vi "Convert To Palette Data.vi"(8 "error in (no error)":errorcluster, 11 "Predicted Data[]":string[](array[string])) -> (0 "error out":errorcluster, 3 "Array":T1[](array[typedef]))   [LabVIEW 2014, in "SmartPalette.lvlib"]
uses:
  SmartPalette.lvlib
  Controls/Palette Data.ctl
  <vilib>/picture/picture.llb/imagedata.ctl
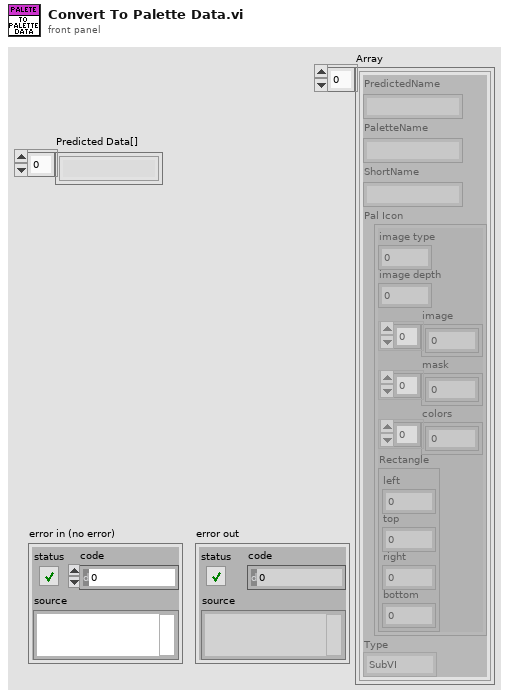
[diagram p1: front panel]
types:
  T1 = typedef "SmartPalette.lvlib/Palette Data.ctl" = cluster{"PredictedName":string, "PaletteName":string, "ShortName":string, "Pal Icon":T2, "Type":enum16{"SubVI", "Function"}}
  T2 = typedef "imagedata.ctl" = cluster{"image type":i32, "image depth":i32, "image":u8[], "mask":u8[], "colors":u32[], "Rectangle":cluster{"left":i16, "top":i16, "right":i16, "bottom":i16}}
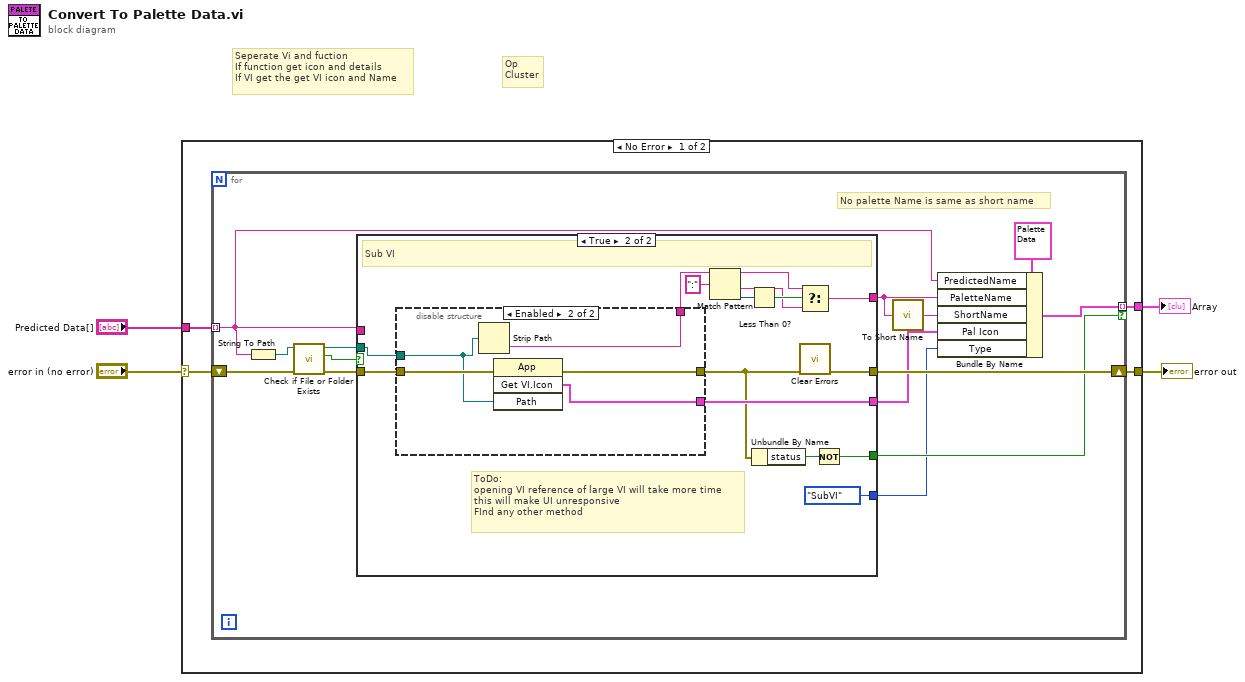
[diagram p0: block diagram]
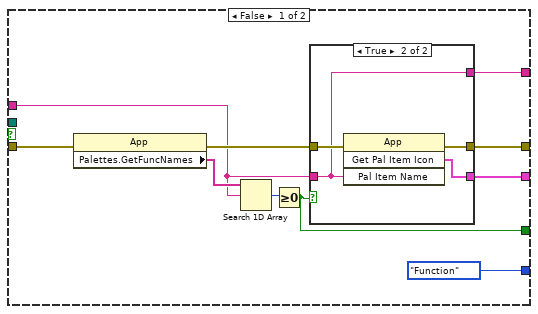
[diagram p2: hidden frame]
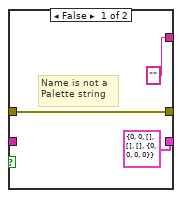
[diagram p3: hidden frame]
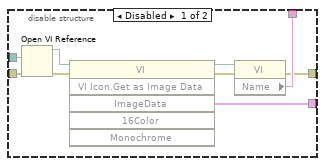
[diagram p4: hidden frame]
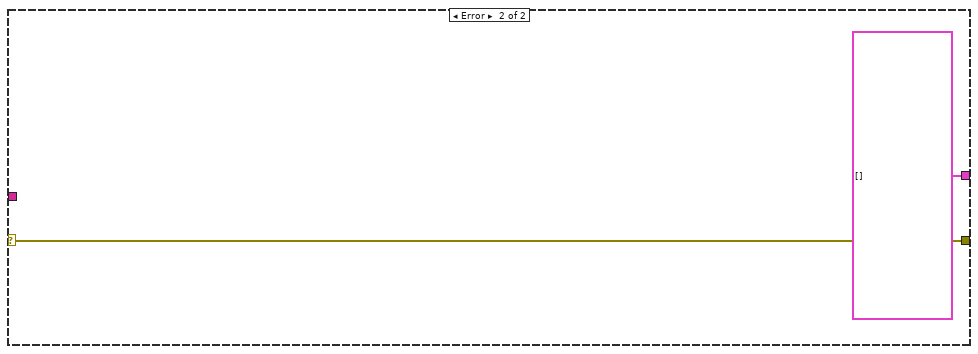
[diagram p5: hidden frame]
diagram:
  # "Op\nCluster"
  # "Seperate Vi and fuction\nIf function get icon and details\nIf VI get the get VI icon and Name"
  n1 = case shown="No Error" "error in (no error)" {
    selector: "error in (no error)" -> [w6 w70]
    tunnel: [w7 w70] -> w3
    tunnel: "Predicted Data[]" -> [w8 _]
    tunnel: [w5 T1[] []] -> w1
    frame No Error {
      n2 = for {
        tunnel: w8 -> [w14] mode=indexing
        shift-right: [w17] -> w7
        shift-left: w6 -> [w22]
        tunnel: [w13] -> w5 mode=indexing if=w12
        # "No palette Name is same as short name"
        n3 = String To Path(string=w14) -> (path=w21:path)
        n4 = call <vilib>:"Check if File or Folder Exists.vi"("error in (no error)"=w22, "path"=w21) -> ("error out"=w18:errorcluster, "file or folder exists?"=w20:bool, "dup path"=w19:path)  [unwired: 7 in]
        n5 = case shown="True" w20 {
          tunnel: w19 -> [_ w53]
          tunnel: w18 -> [w32 w54]
          tunnel: [w28 w41] -> w17
          tunnel: w14 -> [w26 _]
          tunnel: [w27 w52] -> w15
          tunnel: [w25 w45] -> w11
          tunnel: [w24 w42] -> w12
          tunnel: [enum16{"SubVI", "Function"}."Function" ("Type") enum16{"SubVI", "Function"}."SubVI" ("Type")] -> w9
          frame False {
            n6 = property class="App"(error in=w32) -> (error out=w29:errorcluster, "Palettes.GetFuncNames"=w31:string[])  [unwired: 1 in, 1 out]
            n7 = Search 1D Array(1D array=w31, element=w26) -> (index of element=w30:i32)  [unwired: 1 in]
            n8 = Greater Or Equal To 0?(x=w30) -> (x >= 0?=w24:bool)
            n9 = case shown="True" w24 {
              tunnel: w29 -> [w35 w39]
              tunnel: [w35 w38] -> w28
              tunnel: [T2 {"image type"=0, "image depth"=0, "image"=[], "mask"=[], "colors"=[], "Rectangle"={"left"=0, "top"=0, "right"=0, "bottom"=0}} ("Get Pal Item Icon") w37] -> w27
              tunnel: w26 -> [_ w36]
              tunnel: ["" ("String") w36] -> w25
              frame False {
                # "Name is not a \nPalette string"
              }
              frame True {
                n10 = invoke class="App" method="Get Pal Item Icon"(error in=w39, "Pal Item Name"=w36) -> (error out=w38:errorcluster, "Get Pal Item Icon"=w37:T2)  [unwired: 2 in, 2 out]
              }
            }
          }
          frame True {
            # "ToDo:\nopening VI reference of large VI will take more time\nthis will make UI unresponsive \nFInd any other method"
            # "Sub VI"
            n11 = disable-structure shown="Enabled" {
              disable-tunnel: w54 -> [w63 w68]
              disable-tunnel: w53 -> [w61 w65]
              disable-tunnel: [w59 w66] -> w52
              disable-tunnel: [w56 w64] -> w46
              disable-tunnel: [w55 w67] -> w44
              frame Disabled {
                n12 = Open VI Reference(vi path=w61, error in (no error)=w63) -> (vi reference=w60:refnum<vi>, error out=w62:errorcluster)  [unwired: 4 in]
                n13 = invoke class="VI" method="VI Icon.Get as Image Data"(reference=w60, error in=w62) -> (reference out=w57:refnum<vi>, error out=w58:errorcluster, "ImageData"=w59:T2)  [unwired: 4 in, 3 out]
                n14 = property class="VI"(reference=w57, error in=w58) -> (error out=w55:errorcluster, "Name"=w56:string)  [unwired: 1 out]
              }
              frame Enabled {
                n15 = Strip Path(path=w65) -> (name=w64:string)  [unwired: 1 out]
                n16 = invoke class="App" method="Get VI.Icon"(error in=w68, "Path"=w65) -> (error out=w67:errorcluster, "Get VI.Icon"=w66:T2)  [unwired: 2 in, 2 out]
              }
            }
            n17 = Match Pattern(string=w46, regular expression=":") -> (before substring=w48:string, after substring=w47:string, offset past match=w50:i32)  [unwired: 1 in, 1 out]
            n18 = Less Than 0?(x=w50) -> (x < 0?=w49:bool)
            n19 = Unbundle By Name(w44) -> ("status"=w43:bool)
            n20 = Select(t=w48, s=w49, f=w47) -> (s? t:f=w45:string)
            n21 = call <vilib>:"Clear Errors.vi"("error in (no error)"=w44) -> ("error out"=w41:errorcluster)  [unwired: 5 in, 1 out]
            n22 = Not(x=w43) -> (.not. x?=w42:bool)
          }
        }
        n23 = call "To Short Name.vi"("string"=w11) -> ("String out"=w10:string)
        n24 = Bundle By Name(cluster=T1 {"PredictedName"="", "PaletteName"="", "ShortName"="", "Pal Icon"={"image type"=0, "image depth"=0, "image"=[], "mask"=[], "colors"=[], "Rectangle"={"left"=0, "top"=0, "right"=0, "bottom"=0}}, "Type"=enum."SubVI"} ("Palette Data"), "PredictedName"=w14, "PaletteName"=w11, "ShortName"=w10, "Pal Icon"=w15, "Type"=w9) -> (w13:T1)
      }
    }
    frame Error {
    }
  }
  "error out" <- w3
  "Array" <- w1
